vi "Flatten.vi"(8 "error in (no error)":errorcluster, 11 "PC Reader in":refnum<class "PC Reader.lvclass">) -> (0 "error out":errorcluster, 3 "PC Reader out":refnum<class "PC Reader.lvclass">)   [LabVIEW 2017, in "PC Reader.lvclass"]
uses:
  PC Reader.lvclass
  PC Reader.lvclass/PC Reader.ctl
  Global/File Locations.vi
  Reader/Reader.lvclass
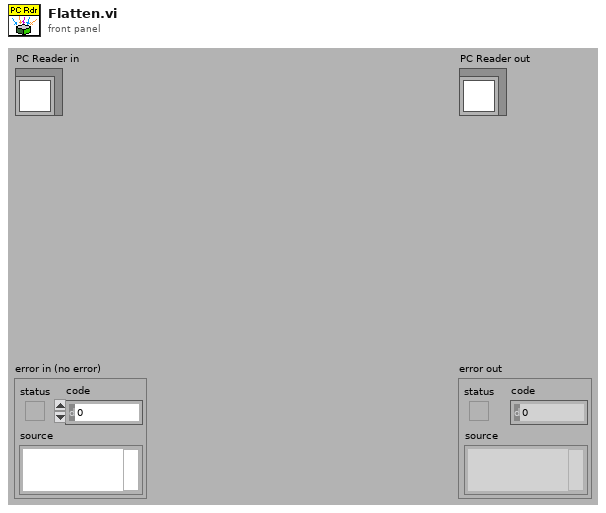
[diagram p1: front panel]
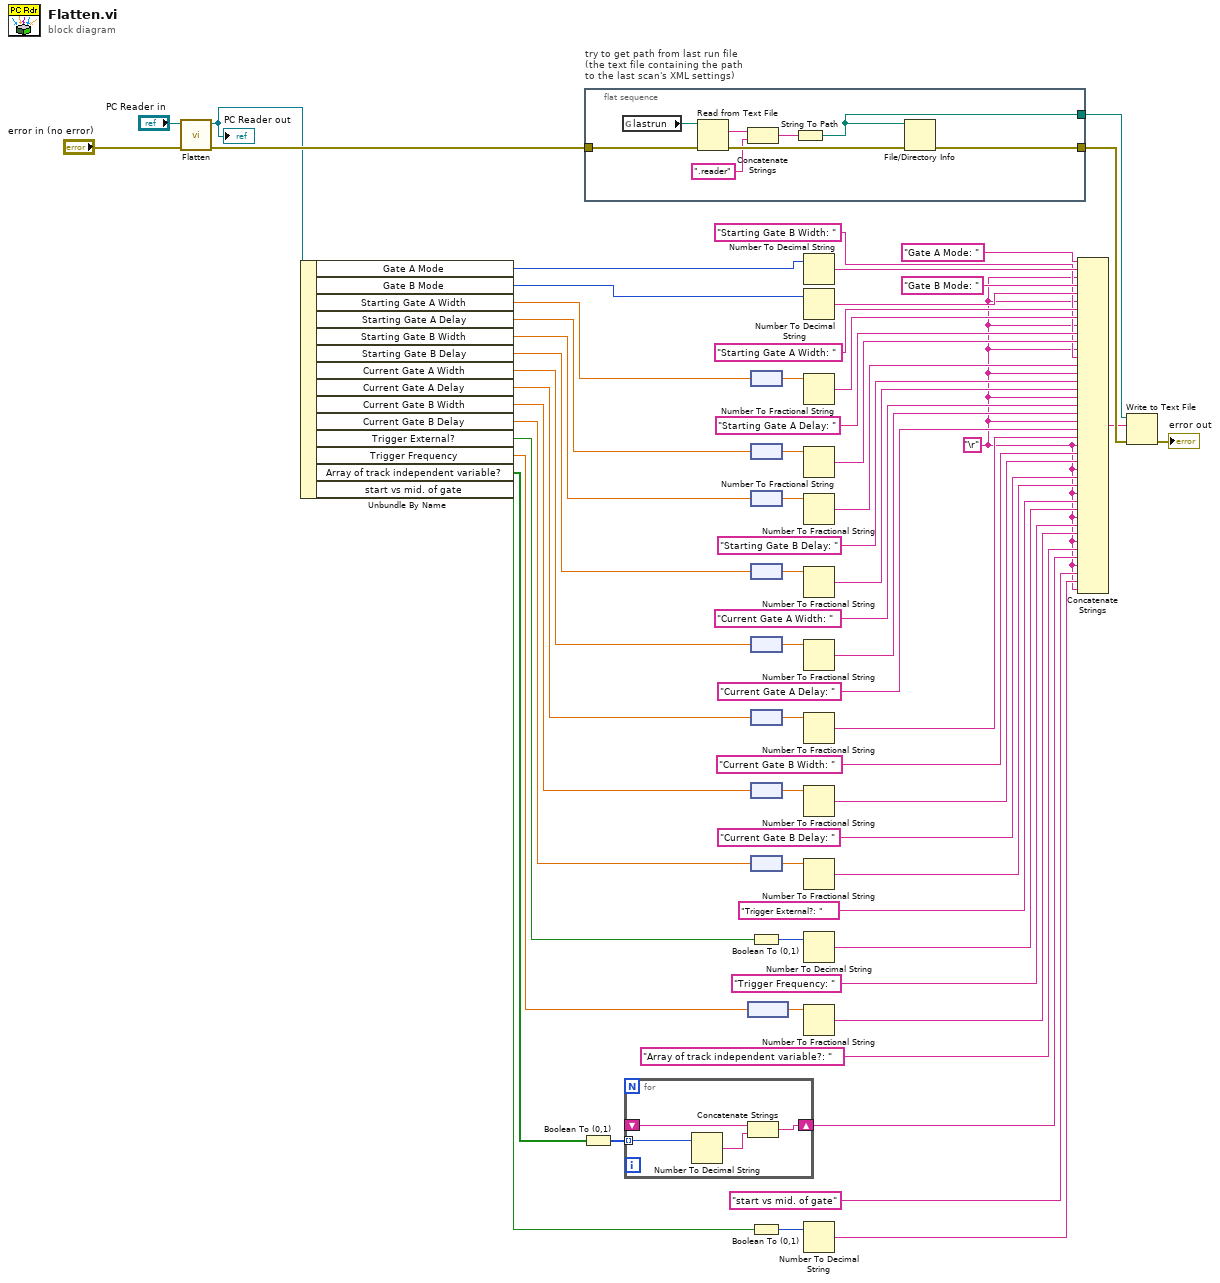
[diagram p0: block diagram]
diagram:
  w2 = "\r"
  n1 = call-parent "Flatten.vi"("error in (no error)"="error in (no error)", "Reader in"="PC Reader in") -> ("error out"=w61:errorcluster, "Reader out"=w57:refnum<class "PC Reader.lvclass">)  [unwired: 8 in]
  "PC Reader out" <- w57
  n2 = Unbundle By Name(w57) -> ("Gate A Mode"=w56:u16, "Gate B Mode"=w55:u16, "Starting Gate A Width"=w50:dbl[unit], "Starting Gate A Delay"=w48:dbl[unit], "Starting Gate B Width"=w46:dbl[unit], "Starting Gate B Delay"=w43:dbl[unit], "Current Gate A Width"=w42:dbl[unit], "Current Gate A Delay"=w39:dbl[unit], "Current Gate B Width"=w38:dbl[unit], "Current Gate B Delay"=w35:dbl[unit], "Trigger External?"=w15:bool, "Trigger Frequency"=w18:dbl[unit], "Array of track independent variable?"=w9:bool[], "start vs mid. of gate"=w4:bool)
  n3 = Boolean To (0,1)(Boolean=w9) -> (0, 1=w8:i16[])
  n4 = flat-sequence "try to get path from last run file\n(the text file containing the path\nto the last scan's XML settings)" {
    tunnel: [w69] -> w59
    tunnel: w61 -> [w68]
    tunnel: [w64] -> w58
    frame #0 {
      n5 = global read "File Locations.vi" "lastrun"() -> (w71:path)
      n6 = Read from Text File(file (use dialog)=w71, error in=w68) -> (text=w67:string, error out=w70:errorcluster)  [unwired: 4 out]
      n7 = Concatenate Strings(w67, ".reader") -> (w65:string)
      n8 = String To Path(string=w65) -> (path=w64:path)
      n9 = File/Directory Info(path=w64, error in=w70) -> (error out=w69:errorcluster)  [unwired: 6 out]
    }
  }
  n10 = for {
    shift-right: [w74] -> w7
    shift-left: _ -> [w75]
    tunnel: w8 -> [w72] mode=indexing
    n11 = Number To Decimal String(number=w72) -> (decimal integer string=w73:string)  [unwired: 1 in]
    n12 = Concatenate Strings(w75, w73) -> (w74:string)
  }
  n13 = node(w18) -> (w17:dbl)
  n14 = node(w50) -> (w49:dbl)
  n15 = node(w48) -> (w47:dbl)
  n16 = node(w46) -> (w45:dbl)
  n17 = node(w43) -> (w44:dbl)
  n18 = node(w42) -> (w41:dbl)
  n19 = node(w39) -> (w40:dbl)
  n20 = node(w38) -> (w37:dbl)
  n21 = node(w35) -> (w36:dbl)
  n22 = Boolean To (0,1)(Boolean=w15) -> (0, 1=w16:i16)
  n23 = Boolean To (0,1)(Boolean=w4) -> (0, 1=w5:i16)
  n24 = Number To Decimal String(number=w56) -> (decimal integer string=w53:string)  [unwired: 1 in]
  n25 = Number To Decimal String(number=w55) -> (decimal integer string=w51:string)  [unwired: 1 in]
  n26 = Number To Fractional String(number=w49) -> (F-format string=w33:string)  [unwired: 3 in]
  n27 = Number To Fractional String(number=w47) -> (F-format string=w31:string)  [unwired: 3 in]
  n28 = Number To Fractional String(number=w45) -> (F-format string=w29:string)  [unwired: 3 in]
  n29 = Number To Fractional String(number=w44) -> (F-format string=w27:string)  [unwired: 3 in]
  n30 = Number To Fractional String(number=w41) -> (F-format string=w25:string)  [unwired: 3 in]
  n31 = Number To Fractional String(number=w40) -> (F-format string=w23:string)  [unwired: 3 in]
  n32 = Number To Fractional String(number=w37) -> (F-format string=w21:string)  [unwired: 3 in]
  n33 = Number To Fractional String(number=w36) -> (F-format string=w19:string)  [unwired: 3 in]
  n34 = Number To Decimal String(number=w16) -> (decimal integer string=w13:string)  [unwired: 1 in]
  n35 = Number To Fractional String(number=w17) -> (F-format string=w11:string)  [unwired: 3 in]
  n36 = Number To Decimal String(number=w5) -> (decimal integer string=w3:string)  [unwired: 1 in]
  n37 = Concatenate Strings("Gate A Mode: ", w53, w2, "Gate B Mode: ", w51, w2, "Starting Gate A Width: ", w33, w2, "Starting Gate A Delay: ", w31, w2, "Starting Gate B Width: ", w29, w2, "Starting Gate B Delay: ", w27, w2, "Current Gate A Width: ", w25, w2, "Current Gate A Delay: ", w23, w2, "Current Gate B Width: ", w21, w2, "Current Gate B Delay: ", w19, w2, "Trigger External?: ", w13, w2, "Trigger Frequency: ", w11, w2, "Array of track independent variable?: ", w7, w2, "start vs mid. of gate", w3, w2) -> (w1:string)
  n38 = Write to Text File(file (use dialog)=w58, text=w1, error in=w59) -> (error out=→"error out":errorcluster)  [unwired: 1 in, 2 out]
